vi "Close.vi"(8 "error in (no error)":errorcluster, 11 "Yokogawa WT2X0 in":refnum<class "Yokogawa WT2X0.lvclass">) -> (0 "error out":errorcluster, 3 "Yokogawa WT2X0 out":refnum<class "Yokogawa WT2X0.lvclass">)   [LabVIEW 2014, in "Generic Power Analyzer.lvlib" / "Yokogawa WT2X0.lvlib" / "Yokogawa WT2X0.lvclass"]
uses:
  Yokogawa WT2X0.lvclass
  <instrlib>/Yokogawa WT200 Series/Yokogawa WT200 Series.lvlib
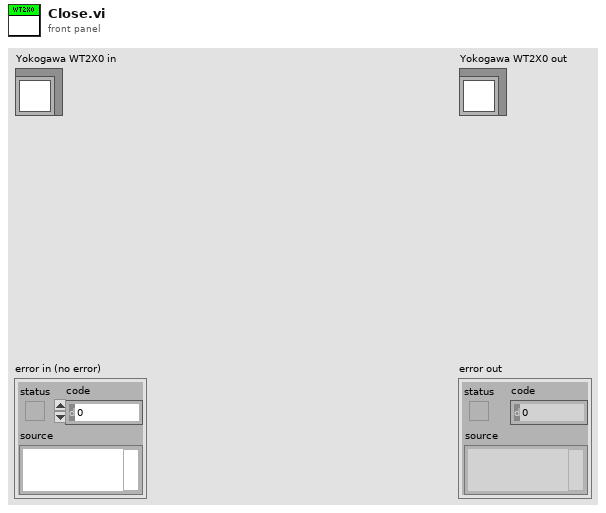
[diagram p1: front panel]
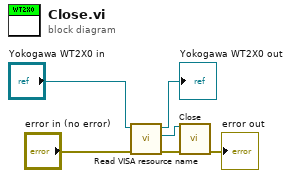
[diagram p0: block diagram]
diagram:
  n1 = call-dynamic "Read VISA resource name.vi"("error in (no error)"="error in (no error)", "Generic Instrument in"="Yokogawa WT2X0 in") -> ("error out"=w2:errorcluster, "VISA resource name"=w3:refnum<visa-resource-name>, "Generic Instrument out"=→"Yokogawa WT2X0 out":refnum<class "Yokogawa WT2X0.lvclass">)  [unwired: 7 in]
  n2 = call <instrlib>:"Close.vi"("VISA resource name"=w3, "error in (no error)"=w2) -> ("error out"=→"error out":errorcluster)  [unwired: 13 in]
